vi "ATCasesTicket.vi"(0 "session in":refnum<k35>, 5 "GEA2 Reference In":refnum<k24>, 7 "Steps":T2(array[cluster])) -> (4 "session out":refnum<k35>, 6 "GEA2 Reference Out":refnum<k24>, 8 "Data Result":T1(array[cluster]))   [LabVIEW 2021]
uses:
  D:/Common/LabVIEW GEA2 Toolkit/source/GEA3 DLL Source/GeaCommunication.dll
  Common/LabVIEW GEA2 Toolkit/source/GEA3 DLL Source/GeaCommunication.dll
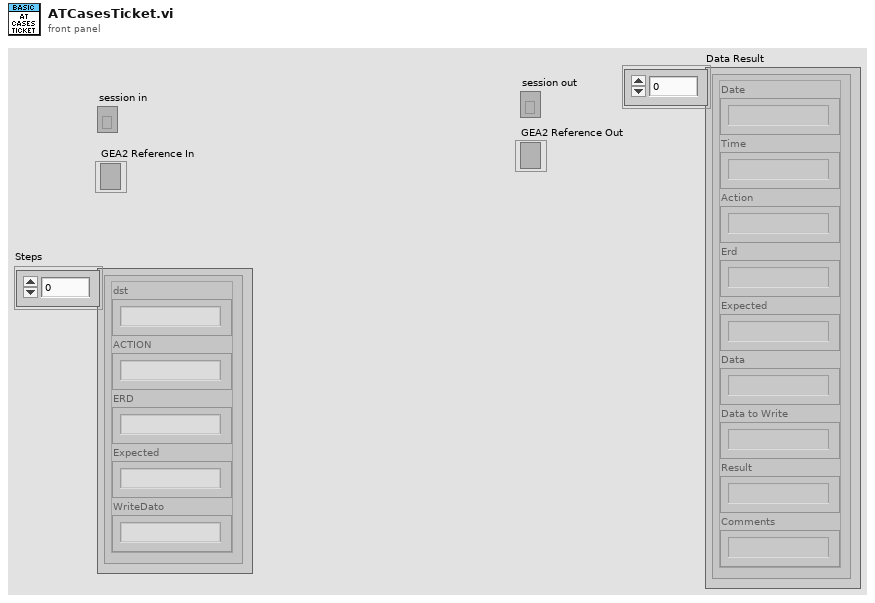
[diagram p1: front panel]
types:
  T1 = cluster{"Date":string, "Time":string, "Action":string, "Erd":string, "Expected":string, "Data":string, "Data to Write":string, "Result":string, "Comments":string}[]
  T2 = cluster{"dst":string, "ACTION":string, "ERD":string, "Expected":string, "WriteDato":string}[]
  T3 = cluster{"Date":string, "Time":string, "Action":string, "Erd":string, "Expected":string, "Data":string, "Data to Write":string, "Result":string, "Comments":string}
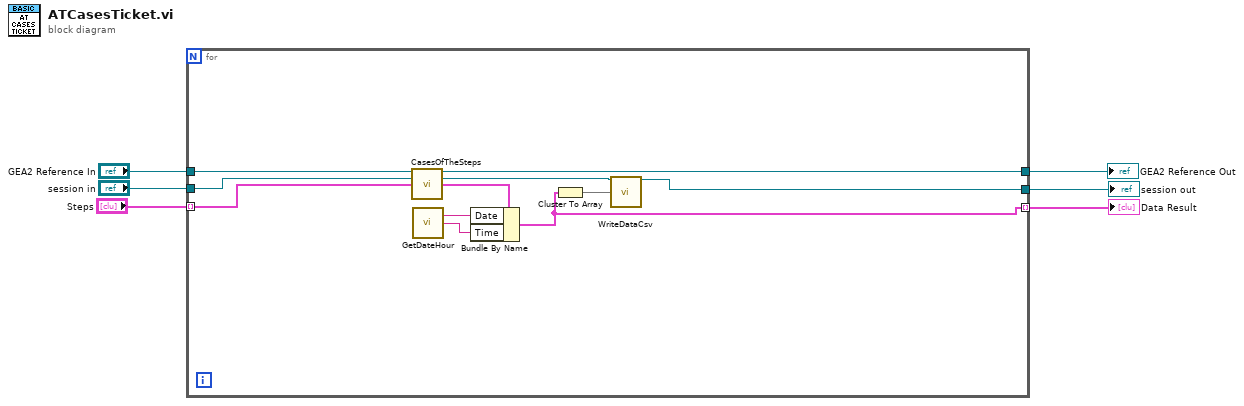
[diagram p0: block diagram]
diagram:
  n1 = for {
    tunnel: "Steps" -> [w15] mode=indexing
    tunnel: "GEA2 Reference In" -> [w17]
    tunnel: [w14] -> w4
    tunnel: "session in" -> [w16]
    tunnel: [w12] -> w2
    tunnel: [w7] -> w1 mode=indexing
    n2 = call "CasesOfTheSteps.vi"("GEA2 Reference In"=w17, "session in"=w16, "Cluster"=w15) -> ("GEA2 Reference Out"=w14:refnum<k24>, "session out"=w13:refnum<k35>, "Results"=w10:T3)  [unwired: 10 in]
    n3 = call "GetDateHour.vi"() -> ("Date"=w8:string, "Hour"=w9:string)  [unwired: 14 in]
    n4 = Bundle By Name(cluster=w10, "Date"=w8, "Time"=w9) -> (w7:T3)
    n5 = Cluster To Array(cluster=w7) -> (array=w11:string[])
    n6 = call "WriteDataCsv.vi"("session in"=w13, "Array Results"=w11) -> ("session out"=w12:refnum<k35>)  [unwired: 12 in, 1 out]
  }
  "GEA2 Reference Out" <- w4
  "session out" <- w2
  "Data Result" <- w1
